vi "Property Names.vi"() -> (3 "Property Names":string[](array[string]))   [LabVIEW 2016, in "Imager Handler.lvclass"]
uses:
  Imager Handler.lvclass
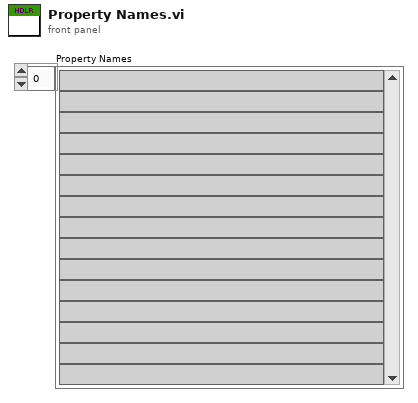
[diagram p1: front panel]
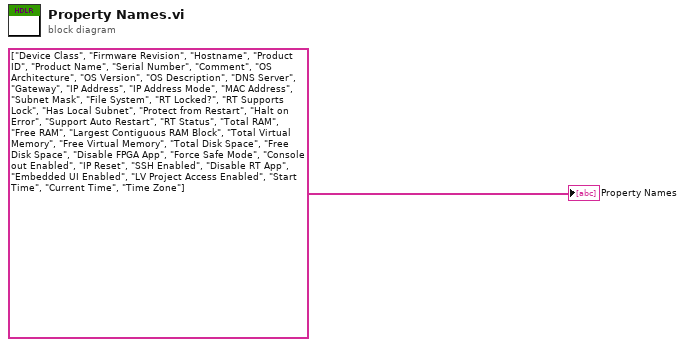
[diagram p0: block diagram]
diagram:
  "Property Names" <- string[] ["Device Class", "Firmware Revision", "Hostname", "Product ID", "Product Name", "Serial Number", "Comment", "OS Architecture", "OS Version", "OS Description", "DNS Server", "Gateway", "IP Address", "IP Address Mode", "MAC Address", "Subnet Mask", "File System", "RT Locked?", "RT Supports Lock", "Has Local Subnet", "Protect from Restart", "Halt on Error", "Support Auto Restart", "RT Status", "Total RAM", "Free RAM", "Largest Contiguous RAM Block", "Total Virtual Memory", "Free Virtual Memory", "Total Disk Space", "Free Disk Space", "Disable FPGA App", "Force Safe Mode", "Console out Enabled", "IP Reset", "SSH Enabled", "Disable RT App", "Embedded UI Enabled", "LV Project Access Enabled", "Start Time", "Current Time", "Time Zone"]
